vi "Init DI DAQ v2.vi"(8 "error in":errorcluster, 10 "DAQChan[]":T1[](array[typedef]), 11 "TaskName":string="AI Task") -> (0 "error out":errorcluster, 3 "DI TaskRef":refnum<k21>)   [LabVIEW 2017]
doc: "Developed by Kevin Thompson\nThompson Engineering, LLC\nkevin@thompsonengineering.net"
uses:
  Digital DAQChan--cluster.ctl
  <vilib>/DAQmx/create/channels.llb/DAQmx Create Channel (DI-Digital Input).vi
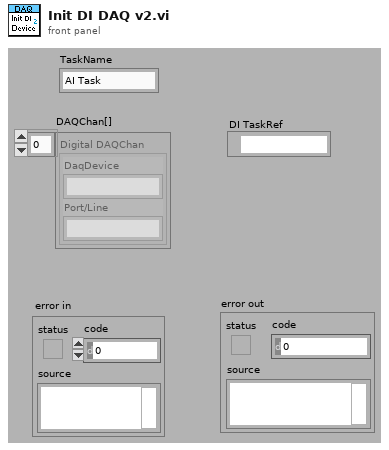
[diagram p1: front panel]
types:
  T1 = typedef "Digital DAQChan--cluster.ctl" = cluster{"DaqDevice":string, "Port/Line":string}
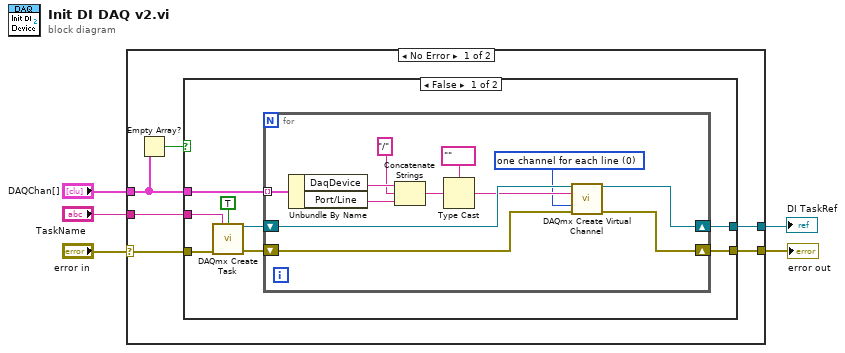
[diagram p0: block diagram]
diagram:
  n1 = case shown="No Error" "error in" {
    selector: "error in" -> [w9 w33]
    tunnel: "DAQChan[]" -> [w6 _]
    tunnel: [w11 _] -> w4
    tunnel: [w10 w33] -> w3
    tunnel: "TaskName" -> [w8 _]
    frame No Error {
      n2 = Empty Array?(array=w6) -> (empty?=w7:bool)
      n3 = case shown="False" w7 {
        tunnel: w6 -> [w19 _]
        tunnel: [w15 _] -> w11
        tunnel: [w14 w32] -> w10
        tunnel: w9 -> [w13 w32]
        tunnel: w8 -> [w12 _]
        frame False {
          n4 = call <vilib>:"DAQmx Create Task.vi"("new task name"=w12, "auto cleanup"=TRUE, "error in"=w13) -> ("task out"=w17:refnum<k21>, "error out"=w16:errorcluster)  [unwired: 11 in]
          n5 = for {
            tunnel: w19 -> [w31] mode=indexing
            shift-right: [w23] -> w15
            shift-left: w17 -> [w25]
            shift-right: [w22] -> w14
            shift-left: w16 -> [w21]
            w20 = 0 items=["one channel for each line", "one channel for all lines"] ("line grouping")
            n6 = Unbundle By Name(w31) -> ("DaqDevice"=w30:string, "Port/Line"=w28:string)
            n7 = Concatenate Strings(w30, "/", w28) -> (w26:string)
            n8 = Type Cast(type=tag "" ("PhysChan"), x=w26) -> (*(type *) &x=w24:tag)
            n9 = call-poly <vilib>:"DAQmx Create Virtual Channel.vi"("task in"=w25, "lines"=w24, "line grouping"=w20, "error in"=w21) -> ("task out"=w23:refnum<k21>, "error out"=w22:errorcluster)  [unwired: 10 in]
          }
        }
        frame True {
        }
      }
    }
    frame Error {
    }
  }
  "DI TaskRef" <- w4
  "error out" <- w3
